vi "PXI-Create DI or DO Tasks.vi"(0 "DAQmx Device Name":tag, 5 "Channel Spec":T2, 7 "Sample Rate":dbl, 9 "Buffer Size":i32, 11 "error in":errorcluster, 12 "Task name":string="DI") -> (4 "Task":T1, 15 "error out":errorcluster)   [LabVIEW 2020]
uses:
  Type Defs/DI Channel Struct.ctl
  Type Defs/Task Struct.ctl
  PXI Globals.vi
  <vilib>/DAQmx/create/channels.llb/DAQmx Create Channel (DI-Digital Input).vi
  <vilib>/DAQmx/create/channels.llb/DAQmx Create Channel (DO-Digital Output).vi
  <vilib>/DAQmx/configure/timing.llb/DAQmx Timing (Sample Clock).vi
  <resource>/objmgr/daqmx.rc
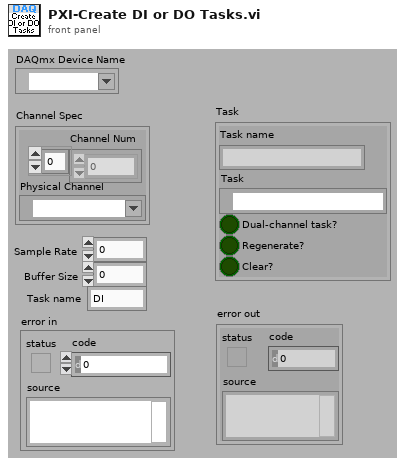
[diagram p1: front panel]
types:
  T1 = typedef "Task Struct.ctl" = cluster{"Task name":string, "Task":refnum<k21>, "Dual-channel task?":bool, "Regenerate?":bool, "Clear?":bool}
  T2 = typedef "DI Channel Struct.ctl" = cluster{"Physical Channel":tag, "Channel Num":i32[]}
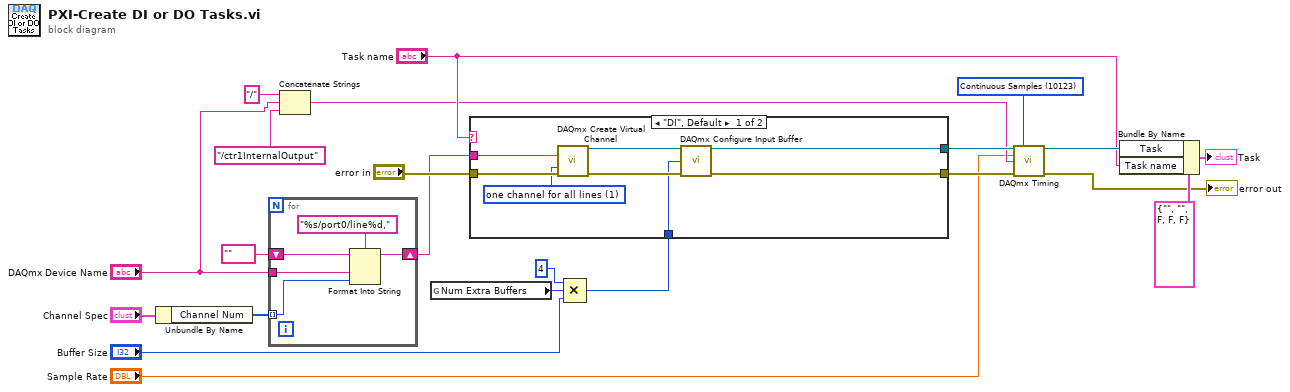
[diagram p0: block diagram]
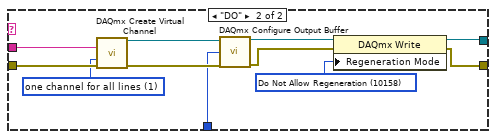
[diagram p2: hidden frame]
diagram:
  w16 = 10123 items=["Finite Samples"=10178, "Continuous Samples"=10123, "Hardware Timed Single Point"=12522] ("sample mode")
  n1 = Unbundle By Name("Channel Spec") -> ("Channel Num"=w18:i32[])
  n2 = for {
    tunnel: w18 -> [w23] mode=indexing
    shift-right: [w25] -> w15
    shift-left: tag "" ("DAQmx Physical Channel") -> [w26]
    tunnel: "DAQmx Device Name" -> [w24]
    n3 = Format Into String(format string="%s/port0/line%d,", initial string=w26, w24, w23) -> (resulting string=w25:string)  [unwired: 1 in, 1 out]
  }
  n4 = Concatenate Strings("/", "DAQmx Device Name", "/ctr1InternalOutput") -> (w3:string)
  n5 = global read "PXI Globals.vi" "Num Extra Buffers"() -> (w13:i32)
  n6 = Compound Arithmetic op=MULTIPLY(4 ("x"), w13, "Buffer Size") -> (w1:i32)
  n7 = case shown="\"DI\", Default" "Task name" {
    tunnel: "error in" -> [w35 w46]
    tunnel: w15 -> [w33 w44]
    tunnel: [w31 w40] -> w5
    tunnel: [w30 w41] -> w4
    tunnel: w1 -> [w28 w38]
    frame "DI", Default {
      w34 = 1 items=["one channel for each line", "one channel for all lines"] ("line grouping")
      n8 = call-poly <vilib>:"DAQmx Create Virtual Channel.vi"("lines"=w33, "line grouping"=w34, "error in"=w35) -> ("task out"=w29:refnum<k21>, "error out"=w32:errorcluster)  [unwired: 11 in]
      n9 = call <vilib>:"DAQmx Configure Input Buffer.vi"("task/channels in"=w29, "buffer size (in samples per channel)"=w28, "error in"=w32) -> ("task out"=w30:refnum<k21>, "error out"=w31:errorcluster)  [unwired: 11 in]
    }
    frame "DO" {
      w39 = 10158 items=["Allow Regeneration"=10097, "Do Not Allow Regeneration"=10158] ("RegenMode")
      w45 = 1 items=["one channel for each line", "one channel for all lines"] ("line grouping")
      n10 = call-poly <vilib>:"DAQmx Create Virtual Channel.vi"("lines"=w44, "line grouping"=w45, "error in"=w46) -> ("task out"=w43:refnum<k21>, "error out"=w42:errorcluster)  [unwired: 11 in]
      n11 = call <vilib>:"DAQmx Configure Output Buffer.vi"("task/channels in"=w43, "buffer size (in samples per channel)"=w38, "error in"=w42) -> ("task out"=w37:refnum<k21>, "error out"=w36:errorcluster)  [unwired: 11 in]
      n12 = property class="DAQmx Write"(reference=w37, error in=w36, "Regeneration Mode"=w39) -> (reference out=w41:refnum<k21>, error out=w40:errorcluster)
    }
  }
  n13 = call-poly <vilib>:"DAQmx Timing.vi"("task/channels in"=w4, "sample mode"=w16, "rate"="Sample Rate", "source"=w3, "error in"=w5) -> ("task out"=w12:refnum<k21>, "error out"=→"error out":errorcluster)  [unwired: 9 in]
  n14 = Bundle By Name(cluster=T1 {"Task name"="", "Task"="", "Dual-channel task?"=FALSE, "Regenerate?"=FALSE, "Clear?"=FALSE} ("Dummy task"), "Task"=w12, "Task name"="Task name") -> (→"Task":T1)
